vi "Anytime D Star Initialize.vi"(6 "manual epsilon (T)":bool=TRUE, 8 "error in (no error)":errorcluster, 9 "goal reference":refnum<data-value>, 10 "start reference":refnum<data-value>, 11 "map reference in":refnum<data-value>) -> (0 "error out":errorcluster, 2 "Anytime D*":refnum<class "NI_Robotics_AnytimeDStar.lvclass">)   [LabVIEW 2017, in "NI_Robotics_AnytimeDStar.lvclass"]
doc: "Initializes a path planning session with which the AD* VI operates."
uses:
  <vilib>/robotics/Navigation/Anytime D Star/NI_Robotics_AnytimeDStar.lvclass
  <vilib>/robotics/Navigation/shared/MapNode/AbstractDstarNode/NI_Robotics_AbstractDstarNode.lvclass
  <vilib>/robotics/Navigation/shared/WorldMap/AbstractDstarWorldMap/NI_Robotics_AbstractDstarWorldMap.lvclass
  <vilib>/robotics/Navigation/shared/Priority Queue/NI_Robotics_Priority Queue.lvclass
  <vilib>/robotics/Navigation/Anytime D Star/NI_Robotics_AnytimeDStar.lvclass/NI_Robotics_AnytimeDStar.ctl
  <vilib>/robotics/Navigation/shared/InconsistentList/NI_Robotics_InconsistentList.lvclass
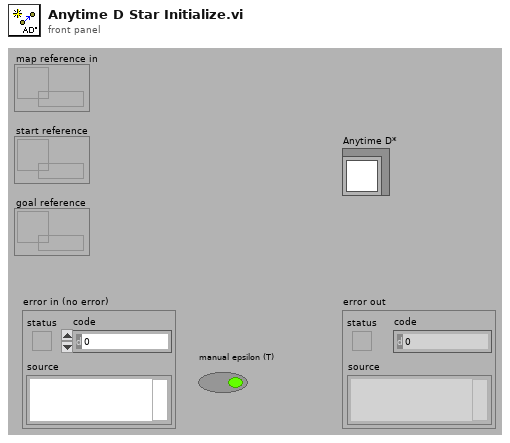
[diagram p1: front panel]
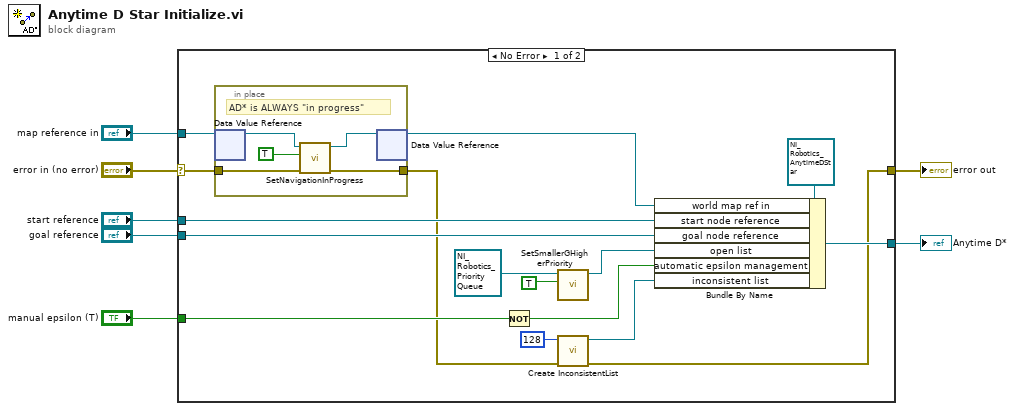
[diagram p0: block diagram]
diagram:
  n1 = case shown="No Error" "error in (no error)" {
    selector: "error in (no error)" -> [w20 w29]
    tunnel: "map reference in" -> [w11 _]
    tunnel: "manual epsilon (T)" -> [w16 _]
    tunnel: [w23 _] -> w5
    tunnel: "start reference" -> [w22 _]
    tunnel: "goal reference" -> [w21 _]
    tunnel: [w9 w29] -> w2
    frame No Error {
      n2 = in-place {
        in-place-border: [w25] -> w8
        in-place-border: w20 -> [w24]
        # "AD* is ALWAYS \"in progress\""
        n3 = in-place-dvr #1(w11) -> (w28:refnum<class "NI_Robotics_AbstractDstarWorldMap.lvclass">)  [unwired: 1 out]
        n4 = call-dynamic "SetNavigationInProgress.vi"("error in (no error)"=w24, "navigation in progress"=TRUE ("Navigation in Progress"), "AbstractWorldMap in"=w28) -> ("error out"=w25:errorcluster, "AbstractWorldMap out"=w26:refnum<class "NI_Robotics_AbstractDstarWorldMap.lvclass">)  [unwired: 7 in]
        n5 = in-place-dvr #1(w26) -> (w10:refnum<data-value>)  [unwired: 1 out]
      }
      n6 = Not(x=w16) -> (.not. x?=w15:bool)
      n7 = call <vilib>:"SetSmallerGHigherPriority.vi"("smaller g = higher priority"=TRUE, "priority queue in"=refnum<class "NI_Robotics_Priority Queue.lvclass"> refnum) -> ("priority queue out"=w18:refnum<class "NI_Robotics_Priority Queue.lvclass">)  [unwired: 9 in]
      n8 = call <vilib>:"Create InconsistentList.vi"("error in (no error)"=w8, "initial allocated size"=128) -> ("error out"=w9:errorcluster, "inconsistent list"=w14:refnum<class "NI_Robotics_InconsistentList.lvclass">)  [unwired: 8 in]
      n9 = Bundle By Name(cluster=refnum<class "NI_Robotics_AnytimeDStar.lvclass"> refnum ("NI_Robotics_AnytimeDStar.lvclass"), "world map ref in"=w10, "start node reference"=w22, "goal node reference"=w21, "open list"=w18, "automatic epsilon management"=w15, "inconsistent list"=w14) -> (w23:refnum<class "NI_Robotics_AnytimeDStar.lvclass">)
    }
    frame Error {
    }
  }
  "Anytime D*" <- w5
  "error out" <- w2
